vi "OFDM_BB_Mod_Demod.vi"() -> ()   [LabVIEW 2009]
uses:
  <vilib>/imath/engines/lvmath2/RunTimeEngine/ErrorHandling/NIMS_Finalize Error.vi
  <vilib>/imath/engines/lvmath2/RunTimeEngine/Parser/MC_Version.vi
  <vilib>/imath/engines/lvmath2/RunTimeEngine/NodeEndStatement/NIMS_NodeEndStatement_Output.vi
  <instcachedir>/0/NIMS_NodeEndStatement_Output_53EC0D466D134D7ABD903AC30B43404B.lvgen/NIMS_NodeEndStatement_Output_53EC0D466D134D7ABD903AC30B43404B_001.vi
  <vilib>/imath/engines/lvmath2/RunTimeEngine/RangeToken/NIMS_Range.vi
  <instcachedir>/0/NIMS_Range_08574DECC23E450FAF0AC0BC39E6BEA7.lvgen/NIMS_Range_08574DECC23E450FAF0AC0BC39E6BEA7_001.vi
  <vilib>/imath/engines/lvmath/Functions/Error Handling/MergeErrorsWrapper.vi
  <vilib>/imathl/engines/lvmath/Functions/Error Handling/Create Error.vi
  <vilib>/imath/engines/lvmath/Functions/Error Handling/MC_Error Cluster From Error Code.vi
  <vilib>/imath/engines/lvmath2/RunTimeEngine/BuiltInFunctions/rand/NIMS_rand(1,I32).vi
  <vilib>/imath/engines/lvmath2/RunTimeEngine/ArithmeticOperatorToken/NIMS_ArithmeticOperator_plus.vi
  <instcachedir>/0/NIMS_ArithmeticOperator_plus_48B9519178ED42D7840F01273E784BFE.lvgen/NIMS_ArithmeticOperator_plus_48B9519178ED42D7840F01273E784BFE_001.vi
  <vilib>/imath/engines/lvmath2/RunTimeEngine/ReplaceToken/NIMS_Replace - M(S)=S.vi
  <instcachedir>/0/NIMS_Replace - M(S)=S_A58FEA22B17C423085E579E5B06C4E0E.lvgen/NIMS_Replace - M(S)=S_A58FEA22B17C423085E579E5B06C4E0E_001.vi
  <vilib>/imath/engines/lvmath2/RunTimeEngine/ReplaceToken/NIMS_Replace - Size Check _(_)=S.vi
  <instcachedir>/0/NIMS_Replace - Size Check _(_)=S_C93E24300E2D4FA1B1057E3B3E42F8F7.lvgen/NIMS_Replace - Size Check _(_)=S_C93E24300E2D4FA1B1057E3B3E42F8F7_003.vi
  <vilib>/imath/engines/lvmath2/RunTimeEngine/ReplaceToken/NIMS_Replace - Check Linear.vi
  <instcachedir>/0/NIMS_Replace - Check Linear_3F5099154F904E698C6642037B8E50AB.lvgen/NIMS_Replace - Check Linear_3F5099154F904E698C6642037B8E50AB_003.vi
  <vilib>/imath/engines/lvmath2/RunTimeEngine/ReplaceToken/NIMS_Replace - V(S)=S.vi
  <instcachedir>/0/NIMS_Replace - V(S)=S_1F711D65782C407D901BB57589CB2660.lvgen/NIMS_Replace - V(S)=S_1F711D65782C407D901BB57589CB2660_001.vi
  <instcachedir>/0/NIMS_Replace - Size Check _(_)=S_C93E24300E2D4FA1B1057E3B3E42F8F7.lvgen/NIMS_Replace - Size Check _(_)=S_C93E24300E2D4FA1B1057E3B3E42F8F7_001.vi
  <instcachedir>/0/NIMS_Replace - Check Linear_3F5099154F904E698C6642037B8E50AB.lvgen/NIMS_Replace - Check Linear_3F5099154F904E698C6642037B8E50AB_004.vi
  <vilib>/imath/engines/lvmath2/RunTimeEngine/VariableToken/Read/NIMS_Get Elements - SorM(_) - Check.vi
  <instcachedir>/0/NIMS_Get Elements - SorM(_) - Check_19F9AFF5C34A45CBABECD1A546CADF04.lvgen/NIMS_Get Elements - SorM(_) - Check_19F9AFF5C34A45CBABECD1A546CADF04_004.vi
  <vilib>/imath/engines/lvmath2/RunTimeEngine/BuiltInFunctions/imag/NIMS_imag(Complex).vi
  <instcachedir>/0/NIMS_imag(Complex)_3180D40D00C843A49C2B33397F857BF3.lvgen/NIMS_imag(Complex)_3180D40D00C843A49C2B33397F857BF3_000.vi
  <vilib>/imath/engines/lvmath2/RunTimeEngine/BuiltInFunctions/fft/NIMS_fft(GV).vi
  <instcachedir>/0/NIMS_fft(GV)_4C6467FC22F84E4BA42517A07EF978B0.lvgen/NIMS_fft(GV)_4C6467FC22F84E4BA42517A07EF978B0_000.vi
  <vilib>/imath/engines/lvmath2/RunTimeEngine/BuiltInFunctions/abs/NIMS_abs(signed).vi
  <instcachedir>/0/NIMS_abs(signed)_C4FCB8E6058B49B797C7C8D53CA5F6EC.lvgen/NIMS_abs(signed)_C4FCB8E6058B49B797C7C8D53CA5F6EC_003.vi
  <instcachedir>/0/NIMS_abs(signed)_C4FCB8E6058B49B797C7C8D53CA5F6EC.lvgen/NIMS_abs(signed)_C4FCB8E6058B49B797C7C8D53CA5F6EC_000.vi
  <vilib>/imath/engines/lvmath2/RunTimeEngine/BuiltInFunctions/ifft/NIMS_ifft(CV).vi
panel:
  out "Magnitude Frequency Spectrum":dbl[](graph)
  out "Received (Q) data":dbl[](graph)
  out "Received (I) data":dbl[](graph)
  in  "N1":dbl=64.0
  out "Q data (Time Domain)":dbl[](graph)
  out "I data (Time Domain)":dbl[](graph)
  out "Q data (Frequency Domain)":dbl[](graph)
  out "I data (Frequency Domain)":dbl[](graph)
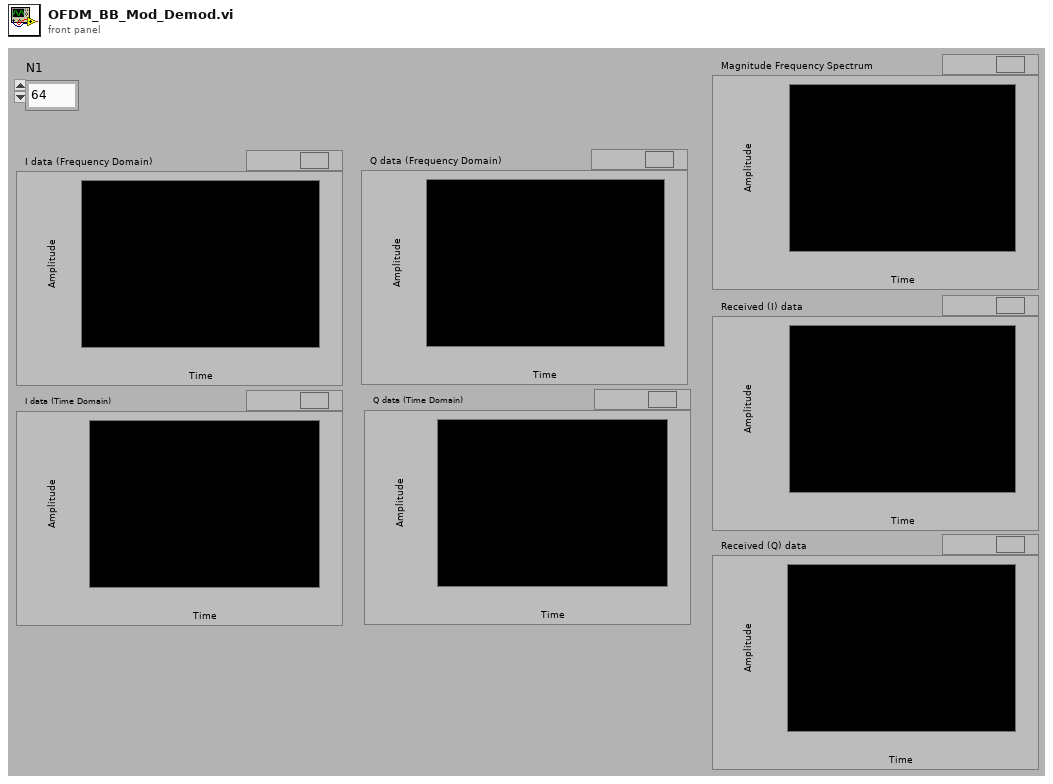
[diagram p1: front panel]
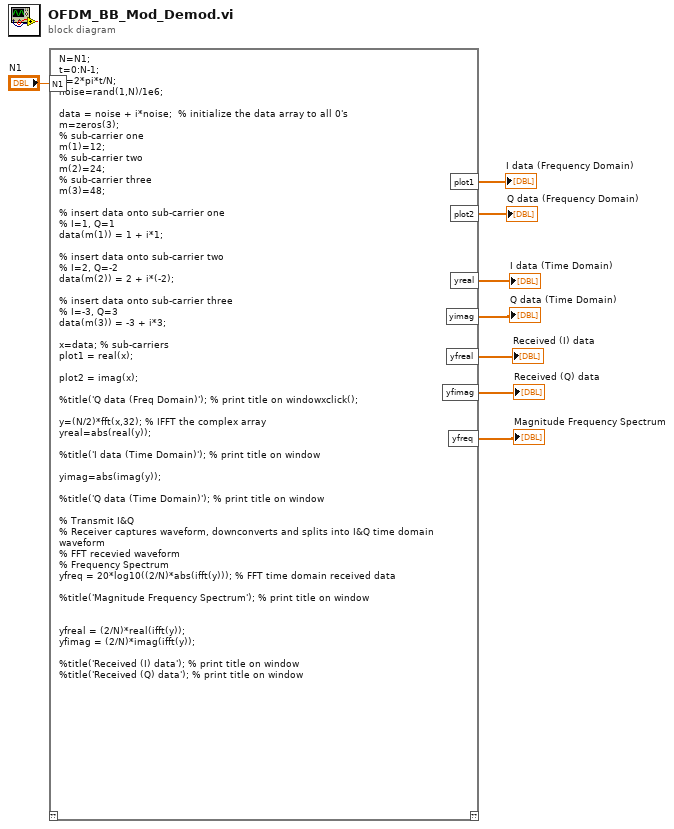
[diagram p0: block diagram]
diagram:
  n1 = mathscript code="N=N1;\nt=0:N-1;\nw=2*pi*t/N;\nnoise=rand(1,N)/1e6;\n\ndata = noise + i*noise;  % initialize the data array to all 0's\nm=zeros(3);\n% sub-carrier one\nm(1)=12;\n% sub-carrier two\nm(2)=24;\n% sub-carrier three\nm(3)=48;\n\n% insert data onto sub-carrier one\n% I=1, Q=1\ndata(m(1)) = 1 + i*1;\n\n% insert data onto sub-carrier two\n% I=2, Q=-2\ndata(m(2)) = 2 + i*(-2);\n\n% insert data onto sub-carrier three\n% I=-3, Q=3\ndata(m(3)) = -3 + i*3;\n\nx=data; % sub-carriers\nplot1 = real(x);\n\nplot2 = imag(x);\n\n%title('Q data (Freq Domain)'); % print title on windowxclick();\n\ny=(N/2)*fft(x,32); % IFFT the complex array\nyreal=abs(real(y));\n\n%title('I data (Time Domain)'); % print title on window\n\nyimag=abs(imag(y));\n\n%title('Q data (Time Domain)'); % print title on window\n\n% Transmit I&Q\n% Receiver captures waveform, downconverts and splits into I&Q time domain waveform\n% FFT recevied waveform\n% Frequency Spectrum\nyfreq = 20*log10((2/N)*abs(ifft(y))); % FFT time domain received data\n\n%title('Magnitude Frequency Spectrum'); % print title on window\n\n\nyfreal = (2/N)*real(ifft(y));\nyfimag = (2/N)*imag(ifft(y));\n\n%title('Received (I) data'); % print title on window\n%title('Received (Q) data'); % print title on window"("N1"="N1") -> ("plot1"=→"I data (Frequency Domain)":dbl[], "plot2"=→"Q data (Frequency Domain)":dbl[], "yreal"=→"I data (Time Domain)":dbl[], "yimag"=→"Q data (Time Domain)":dbl[], "yfreal"=→"Received (I) data":dbl[], "yfimag"=→"Received (Q) data":dbl[], "yfreq"=→"Magnitude Frequency Spectrum":dbl[])  [unwired: 1 in, 1 out]
